vi "execution class name.vi"(8 "error in":errorcluster, 11 "configuration in":refnum<class "PL_Target Configuration.lvclass">) -> (0 "error out":errorcluster, 2 "execution class":string, 3 "configuration out":refnum<class "PL_Target Configuration.lvclass">)   [LabVIEW 2013, in "PL_Target Configuration.lvclass"]
uses:
  PL_Target Configuration.lvclass
  PL_Target Configuration.lvclass/PL_Target Configuration.ctl
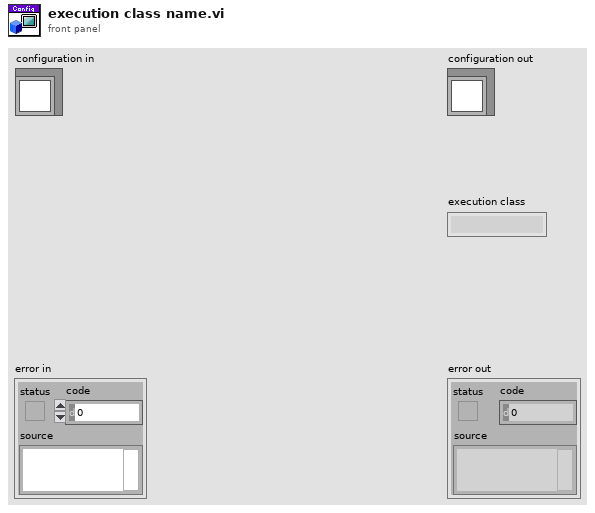
[diagram p1: front panel]
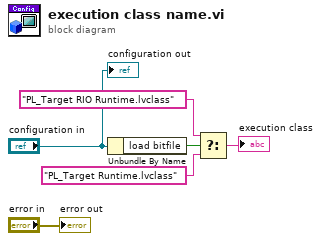
[diagram p0: block diagram]
diagram:
  n1 = Unbundle By Name("configuration in") -> ("load bitfile"=w4:bool)
  n2 = Select(t="PL_Target RIO Runtime.lvclass" ("class name"), s=w4, f="PL_Target Runtime.lvclass" ("class name")) -> (s? t:f=→"execution class":string)
  "error out" <- "error in"
  "configuration out" <- "configuration in"
